vi "Wait_Actor_Test.vi"(8 "error in (no error)":errorcluster caption="entrée d'erreur (pas d'erreur)", 11 "Test (Default) en entrée":refnum<class "Actor Test (Default).lvclass">) -> (0 "error out":errorcluster caption="sortie d'erreur", 3 "Test (Default) en sortie":refnum<class "Actor Test (Default).lvclass">)   [LabVIEW 2020, in "Library Core.lvlib" / "Actor Test (Default).lvclass"]
uses:
  Actor Test (Default).lvclass
  Actor Test (Default).lvclass/Actor Test (Default).ctl
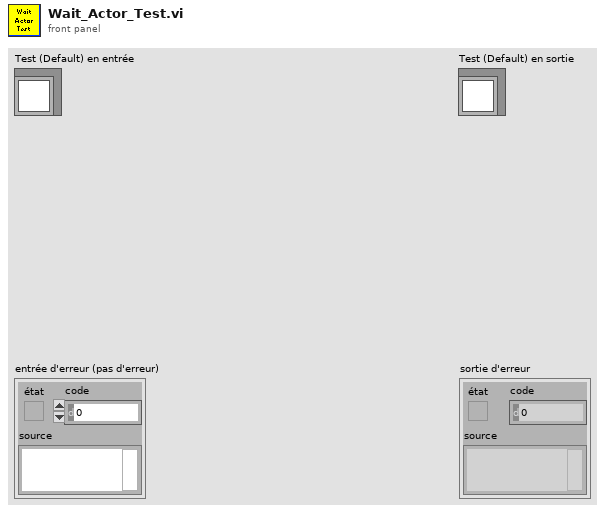
[diagram p1: front panel]
types:
  T1 = typedef "Library Commun.lvlib/Commande Value Type.ctl" = enum16{"None", "String", "Number", "Timestamp", "Boolean", "Array"}
  T2 = typedef "Library Commun.lvlib/Commande Type Test.ctl" = enum16{"Function", "Test", "Calculation"}
  T3 = cluster{"Main Test":string, "Name Test":string, "StartOfTest":string, "Value":string, "Limit_Low":string, "Limit_High":string, "Result":bool, "Fatal_Test":bool, "NbRetry":dbl, "EndOfTest":string, "Error":string, "TypeValue":T1, "Type Test":T2}[]
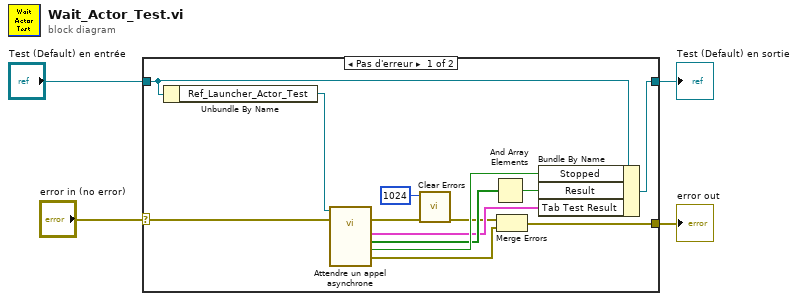
[diagram p0: block diagram]
diagram:
  n1 = case shown="Pas d'erreur" "error in (no error)" {
    selector: "error in (no error)" -> [w5 w19]
    tunnel: [w10 w19] -> w2
    tunnel: [w17 w18] -> w1
    tunnel: "Test (Default) en entrée" -> [w16 w18]
    frame No Error {
      n2 = Unbundle By Name(w16) -> ("Ref_Launcher_Actor_Test"=w6:refnum<vi>)
      n3 = call-by-ref "Attendre un appel asynchrone"(reference=w6, error in=w5) -> (error out=w9:errorcluster, 0:"error out"=w15:errorcluster, "Stopped"=w14:bool, "Results"=w13:bool[], "Tableau"=w11:T3)  [unwired: 8 in, 1 out]
      n4 = call <vilib>:"Clear Errors.vi"("error in (no error)"=w9, "specific error code to clear (0: all)"=1024) -> ("error out"=w8:errorcluster)  [unwired: 4 in, 1 out]
      n5 = And Array Elements(Boolean array=w13) -> (logical AND=w12:bool)
      n6 = Merge Errors(w8, w15) -> (w10:errorcluster)
      n7 = Bundle By Name(cluster=w16, "Stopped"=w14, "Result"=w12, "Tab Test Result"=w11) -> (w17:refnum<class "Actor Test (Default).lvclass">)
    }
    frame Error {
    }
  }
  "error out" <- w2
  "Test (Default) en sortie" <- w1
